vi "initialize.vi"(0 "HGF_Agent":refnum<class "MoAgSy_AgentBase.lvclass">, 3 "initializationData":variant, 5 "error in (no error)":errorcluster, 7 "binaryString":string, 8 "I8 Array":i8[](array[numeric]), 9 "prependSize? (T)":bool, 11 "byteOrder (0:big-endian, network order)":T1(ring)) -> (14 "dup HGF_Agent":refnum<class "MoAgSy_AgentBase.lvclass">, 17 "found?":bool, 19 "error out":errorcluster)   [LabVIEW 2009, in "MoAgSy_Base.lvlib" / "MoAgSy_AgentBase.lvclass"]
doc: "This is a dynamic dispatch VI to be implemented by child classes to initialize their attributes.\n\n<B>Recommendation:</B> Use Variant for initialization data."
uses:
  MoAgSy_AgentBase.lvclass
  MoAgSy_GPG/MoAgSy_GPG.lvclass
  Visitors/MoAgSy_Visitor/MoAgSy_Visitor.lvclass
  HGF_BaseClasses/HGF_Visitable/HGF_Visitable.lvclass
  MoAgSy_AgentBase.lvclass/MoAgSy_AgentBase.ctl
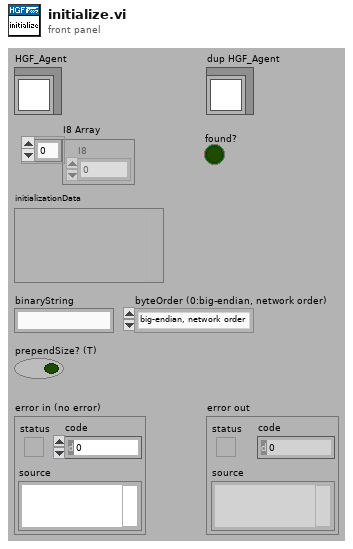
[diagram p1: front panel]
types:
  T1 = enum16{"big-endian, network order", "native, host order", "little-endian"}
  T2 = cluster{"Standard Visitor":refnum<class "MoAgSy_Visitor.lvclass">, "timeout":dbl}
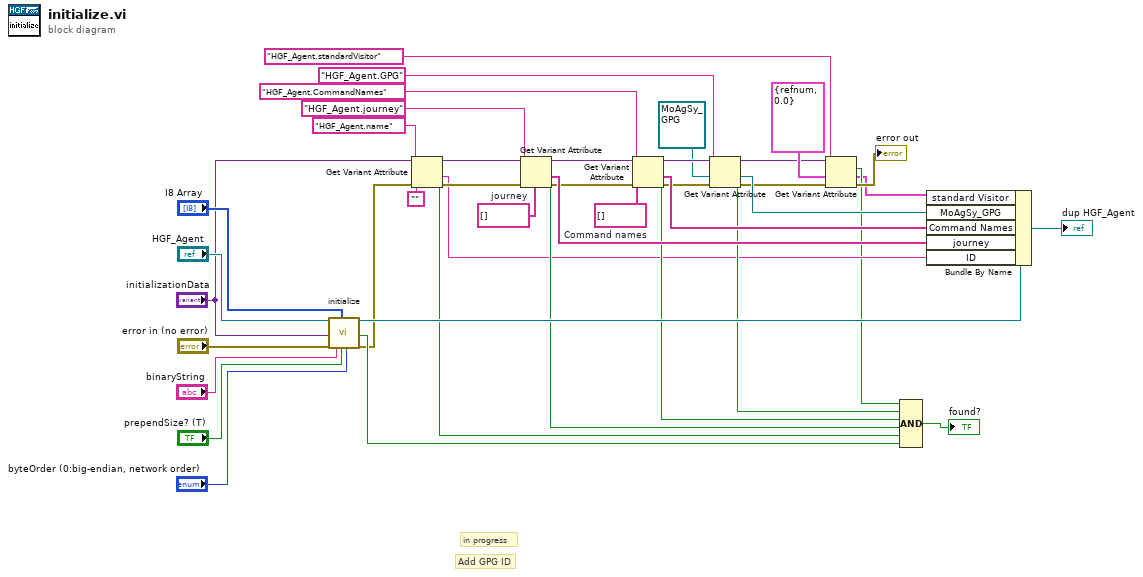
[diagram p0: block diagram]
diagram:
  w17 = string[] []  # journey
  w18 = string[] []  # Command names
  # "Add GPG ID"
  # "in progress"
  n1 = call-parent "initialize.vi"("HGF_Base"="HGF_Agent", "initializationData"="initializationData", "error in (no error)"="error in (no error)", "binaryString"="binaryString", "I8 Array"="I8 Array", "prependSize? (T)"="prependSize? (T)", "byteOrder (0:big-endian, network order)"="byteOrder (0:big-endian, network order)") -> ("dup HGF_Base"=w34:refnum<class "MoAgSy_AgentBase.lvclass">, "found?"=w30:bool, "error out"=w26:errorcluster)  [unwired: 10 out]
  n2 = Get Variant Attribute(Variant="initializationData", name="HGF_Agent.name", default value (empty Variant)="", error in=w26) -> (duplicate Variant=w24:variant, found=w29:bool, value=w8:string, error out=w22:errorcluster)
  n3 = Get Variant Attribute(Variant=w24, name="HGF_Agent.journey", default value (empty Variant)=w17, error in=w22) -> (duplicate Variant=w23:variant, found=w16:bool, value=w41:string[], error out=w21:errorcluster)
  n4 = Get Variant Attribute(Variant=w23, name="HGF_Agent.CommandNames", default value (empty Variant)=w18, error in=w21) -> (duplicate Variant=w13:variant, found=w15:bool, value=w40:string[], error out=w14:errorcluster)
  n5 = Get Variant Attribute(Variant=w13, name="HGF_Agent.GPG", default value (empty Variant)=refnum<class "MoAgSy_GPG.lvclass"> refnum ("MoAgSy.lvlib:MoAgSy_GPG.lvclass"), error in=w14) -> (duplicate Variant=w4:variant, found=w9:bool, value=w10:refnum<class "MoAgSy_GPG.lvclass">, error out=w7:errorcluster)
  n6 = Get Variant Attribute(Variant=w4, name="HGF_Agent.standardVisitor", default value (empty Variant)=T2 {"Standard Visitor"=refnum, "timeout"=0.0} ("standard Visitor"), error in=w7) -> (found=w3:bool, value=w2:T2, error out=→"error out":errorcluster)  [unwired: 1 out]
  n7 = Compound Arithmetic op=AND(w3, w9, w15, w16, w29, w30) -> (→"found?":bool)
  n8 = Bundle By Name(cluster=w34, "standard Visitor"=w2, "MoAgSy_GPG"=w10, "Command Names"=w40, "journey"=w41, "ID"=w8) -> (→"dup HGF_Agent":refnum<class "MoAgSy_AgentBase.lvclass">)
